vi "ngi get dataset secure autostart.vi"(4 "mac adresses":T1, 5 "Auto download":bool, 8 "error in (no error)":errorcluster, 10 "event to file?":bool[](array[boolean]), 11 "Skredhendelser":T2(array[cluster]) {"Intensitet terskel 1" format="%.1f"; "Intensitet terskel 2" format="%.1f"; "Intensitet terskel 3" format="%.1f"; "Intensitet terskel 4" format="%.1f"; "Intensitet terskel 5" format="%.1f"}) -> (0 "error out":errorcluster)   [LabVIEW 2017]
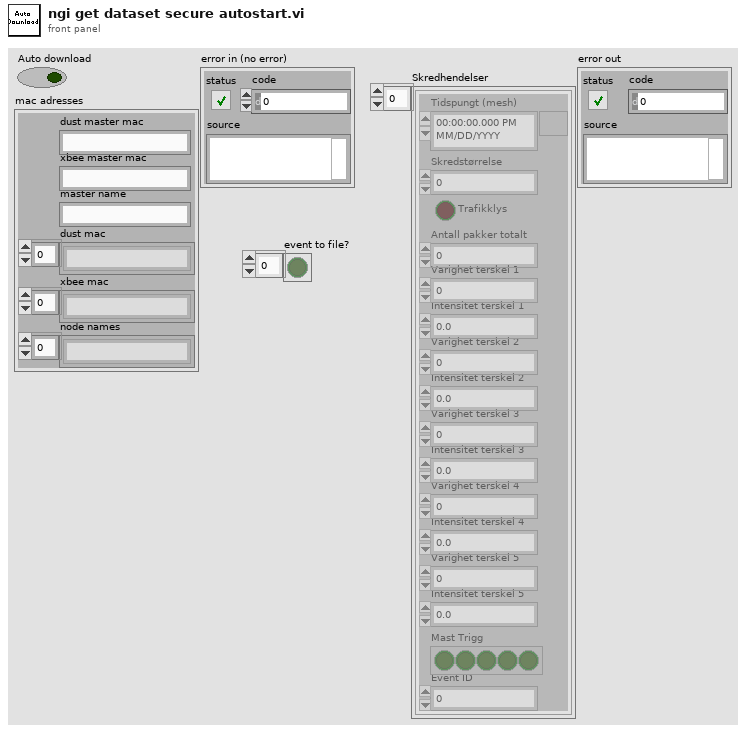
[diagram p1: front panel]
types:
  T1 = cluster{"dust master mac":string, "xbee master mac":string, "master name":string, "dust mac":string[], "xbee mac":string[], "node names":string[]}
  T2 = cluster{"Tidspungt (mesh)":timestamp, "Skredstørrelse":u16, "Trafikklys":bool, "Antall pakker totalt":u16, "Varighet terskel 1":u16, "Intensitet terskel 1":dbl, "Varighet terskel 2":u16, "Intensitet terskel 2":dbl, "Varighet terskel 3":u16, "Intensitet terskel 3":dbl, "Varighet terskel 4":u16, "Intensitet terskel 4":dbl, "Varighet terskel 5":u16, "Intensitet terskel 5":dbl, "Mast Trigg":bool[], "Event ID":i32}[]
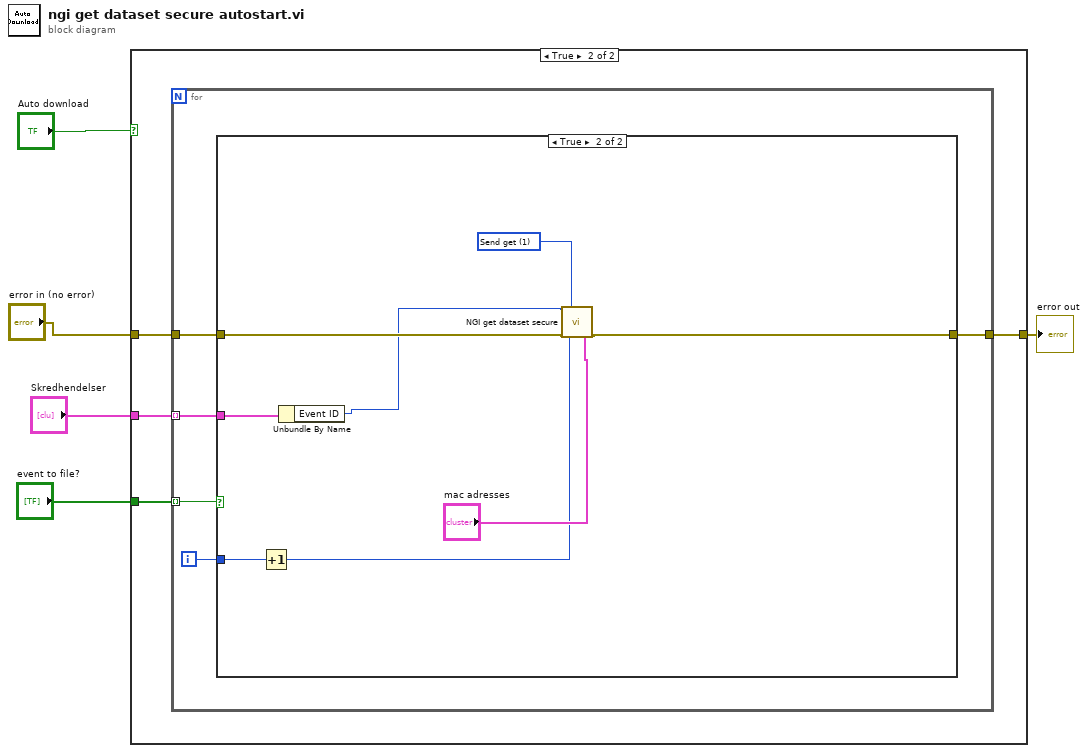
[diagram p0: block diagram]
diagram:
  n1 = case shown="True" "Auto download" {
    tunnel: "event to file?" -> [_ w10]
    tunnel: "Skredhendelser" -> [_ w9]
    tunnel: "error in (no error)" -> [w6 w8]
    tunnel: [w6 w7] -> w1
    frame False {
    }
    frame True {
      n2 = for {
        tunnel: w10 -> [w15] mode=indexing
        tunnel: w9 -> [w14] mode=indexing
        tunnel: w8 -> [w13]
        tunnel: [w12] -> w7
        i -> [w11]
        n3 = case shown="True" w15 {
          tunnel: w14 -> [_ w24]
          tunnel: w13 -> [w16 w20]
          tunnel: [w16 w21] -> w12
          tunnel: w11 -> [_ w23]
          frame False {
          }
          frame True {
            w18 = u16 1 items=["Init array", "Send get", "recive data", "abort secure download"] ("State")
            n4 = Increment(x=w23) -> (x+1=w17:i32)
            n5 = Unbundle By Name(w24) -> ("Event ID"=w19:i32)
            n6 = call "NGI get dataset secure.vi"("ID"=w19, "error in (no error)"=w20, "State"=w18, "Node"=w17, "mac adresses"="mac adresses") -> ("error out"=w21:errorcluster)  [unwired: 11 in, 3 out]
          }
        }
      }
    }
  }
  "error out" <- w1
